vi "Current Loop 9505 (RT).vi"() -> ()   [LabVIEW 2012]
uses:
  <vilib>/LabVIEW Targets/FPGA/cRIO/cRIO-9505/controls.llb/_nicrio_cRIO-9505_DriveStatus.ctl
  <vilib>/addons/control/pid/pid.llb/PID (DBL).vi
  <vilib>/FPGAPlugInAG/cRIO-9074/niLvFpga_Open_cRIO-9074.vi
  <vilib>/Utility/error.llb/Error Cluster From Error Code.vi
  <vilib>/rvi/errors/niLvFpgaAdjustHostInterfaceError.vi
  <vilib>/FPGAPlugInAG/cRIO-9074/niLvFpga_Close_cRIO-9074.vi
  <vilib>/rvi/interface/nirviOpenFPGA/nirviOpenFPGA.xnode
  FPGA Bitfiles/DepthCtrlExperim_FPGATarget_CurrentLoop9505(_EF930710.lvbitx
  <vilib>/rvi/interface/nirviReadWriteControl/nirviReadWriteControl.xnode
  <vilib>/rvi/interface/nirviCloseFPGA/nirviCloseFPGA.xnode
  NiFpgaLv.dll
  <vilib>/addons/control/pid/NI_PID_pid.lvlib
panel:
  out "Time Response":cluster{"Actual Depth (m)":dbl, "setpoint":dbl}(graph)
  out "dt out (s)":dbl
  in  "Reinitialize? (F)":bool
  in  "output range":cluster{"output high":dbl, "output low":dbl}={"output high"=100.0, "output low"=-100.0}
  out "Ctrl Output":dbl
  in  "Sampling Time dt (s)":dbl
  in  "PID gains":T1={"proportional gain (Kc)"=1.0, "integral time (Ti, min)"=0.01, "derivative time (Td, min)"=0.0}
  in  "setpoint":dbl
  in  "Disable":bool
  in  "Disable":bool
  out "Loop Counter DEBUG":dbl
  out "Actual Depth DEBUG":dbl
  in  "Stop AutoTune":bool
  out "Actual Depth (m)":dbl(slide)
  in  "Switch To Autotune Output":bool
  in  "Enable":bool
  in  "Enable":bool
  out "Drive Status 2":T2
  out "Measured Current (Amps) 2":dbl
  in  "Current Loop Rate (usec) 2":u32=50
  in  "Drive Direction 2":enum16{"Clockwise", "Counterclockwise"}(ring)
  in  "Current Setpoint (Amps) 2":dbl(slide)
  in  "Current PI Gains 2":T3={"Proportional Gain"=20, "Integral Gain"=10, "Derivative Gain"=0}
  in  "Current Limit (Amps) 2":dbl=1.0
  in  "Current Limit (Amps)":dbl=1.0
  in  "Current PI Gains":T3={"Proportional Gain"=20, "Integral Gain"=10, "Derivative Gain"=0}
  in  "Current Setpoint (Amps)":dbl(slide)
  out "Measured Current (Amps)":dbl
  out "Drive Status":T2
  in  "Drive Direction":enum16{"Clockwise", "Counterclockwise"}(ring)
  in  "Current Loop Rate (usec)":u32=50
  in  "?":bool
  out "Raw Voltage":dbl(graph)
  out "error out 2":errorcluster
  in  "Wait ms":dbl
  in  "Density of Water":dbl
  in  "Atm Offset":dbl
  out "PSI":dbl(knob)
  out "PSI":dynamicdata(graph)
  out "Absolute Depth (m)":dbl(slide)
  in  "resource name":tag="RIO0::INSTR"
  out "error out":errorcluster
  in  "stop":bool
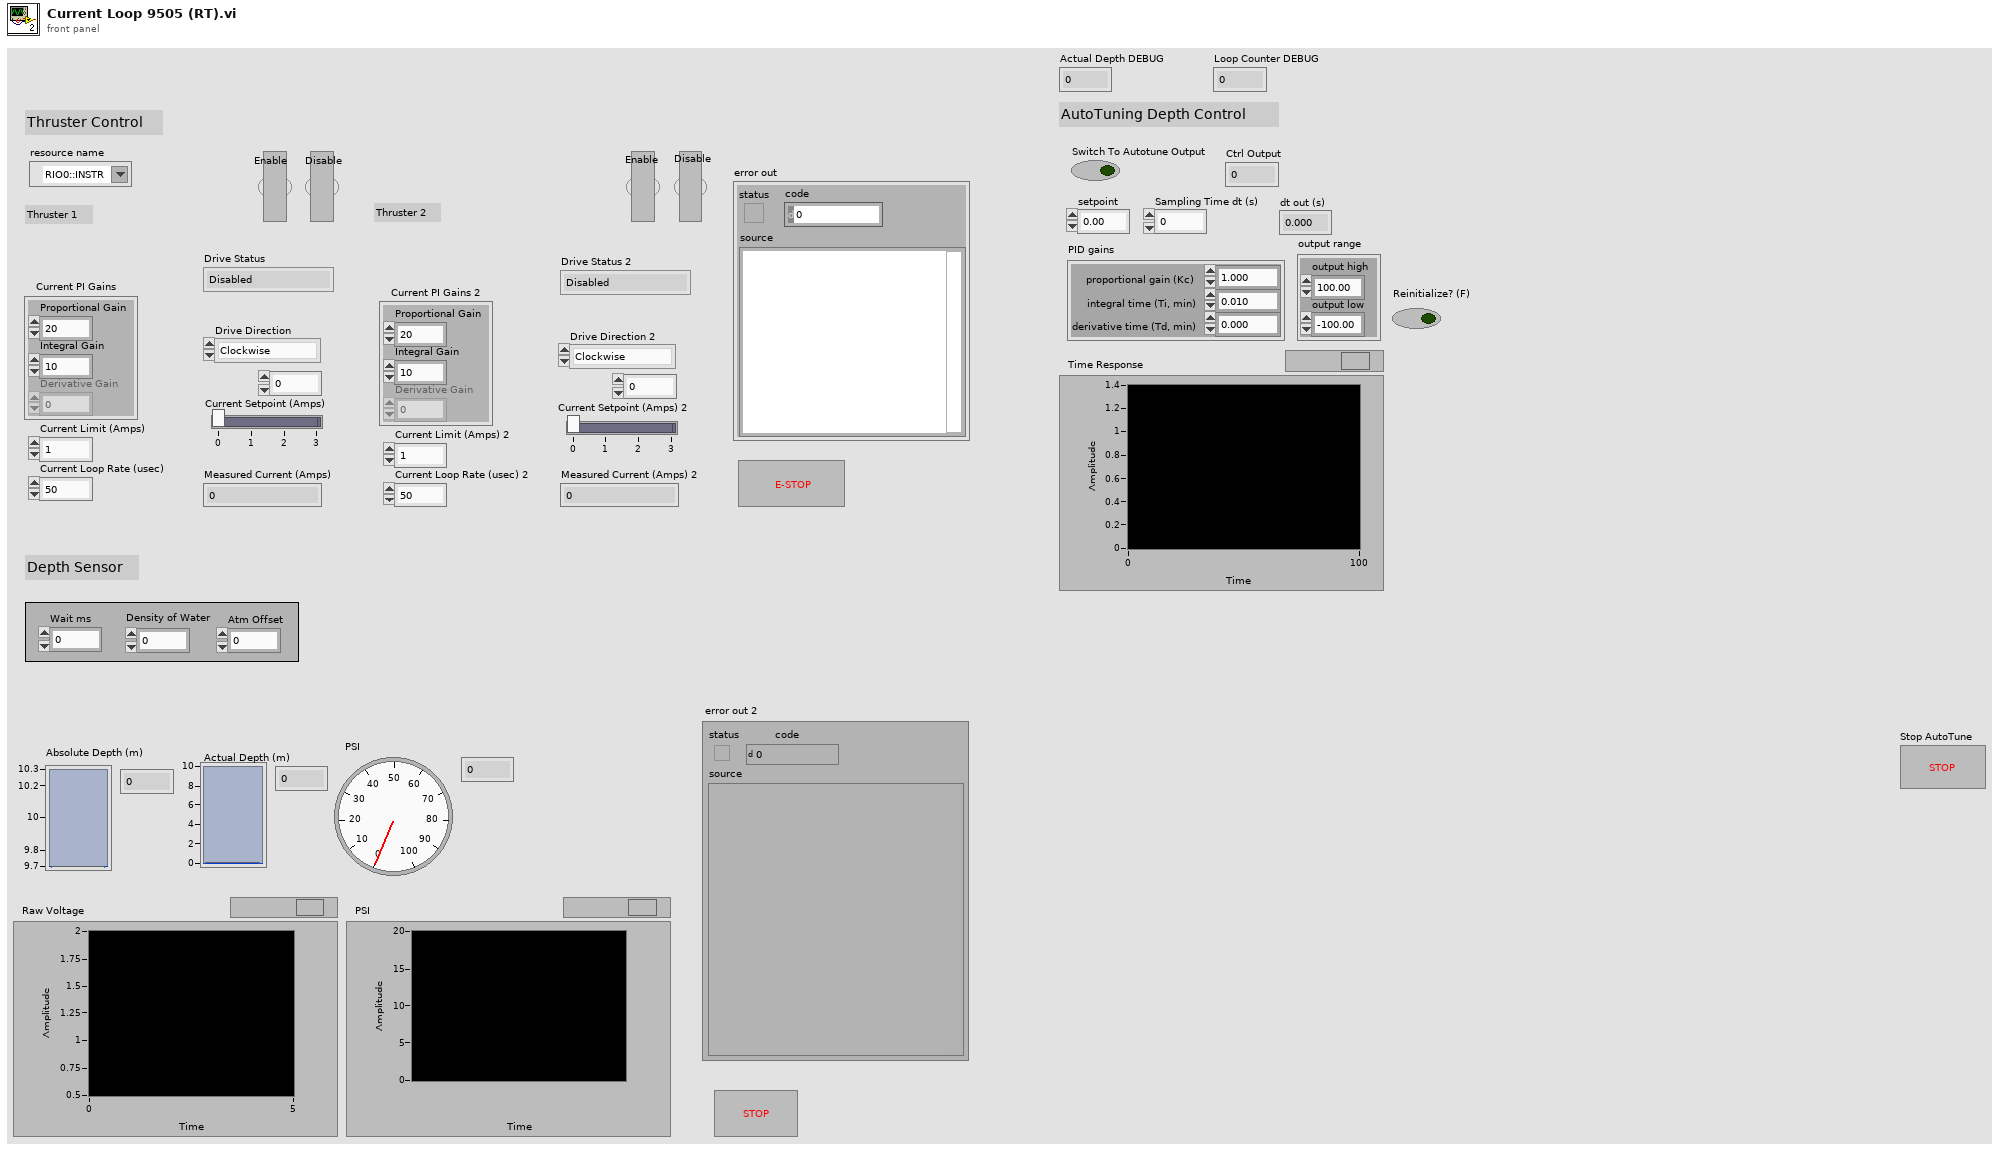
[diagram p1: front panel]
types:
  T1 = cluster{"proportional gain (Kc)":dbl, "integral time (Ti, min)":dbl, "derivative time (Td, min)":dbl}
  T2 = typedef "_nicrio_cRIO-9505_DriveStatus.ctl" = enum8{"Enabled", "Disabled", "Disabled by Drive Fault", "Disabled by Temp. Fault", "Disabled by E-Stop", "Unknown"}
  T3 = cluster{"Proportional Gain":i16, "Integral Gain":i16, "Derivative Gain":i16}
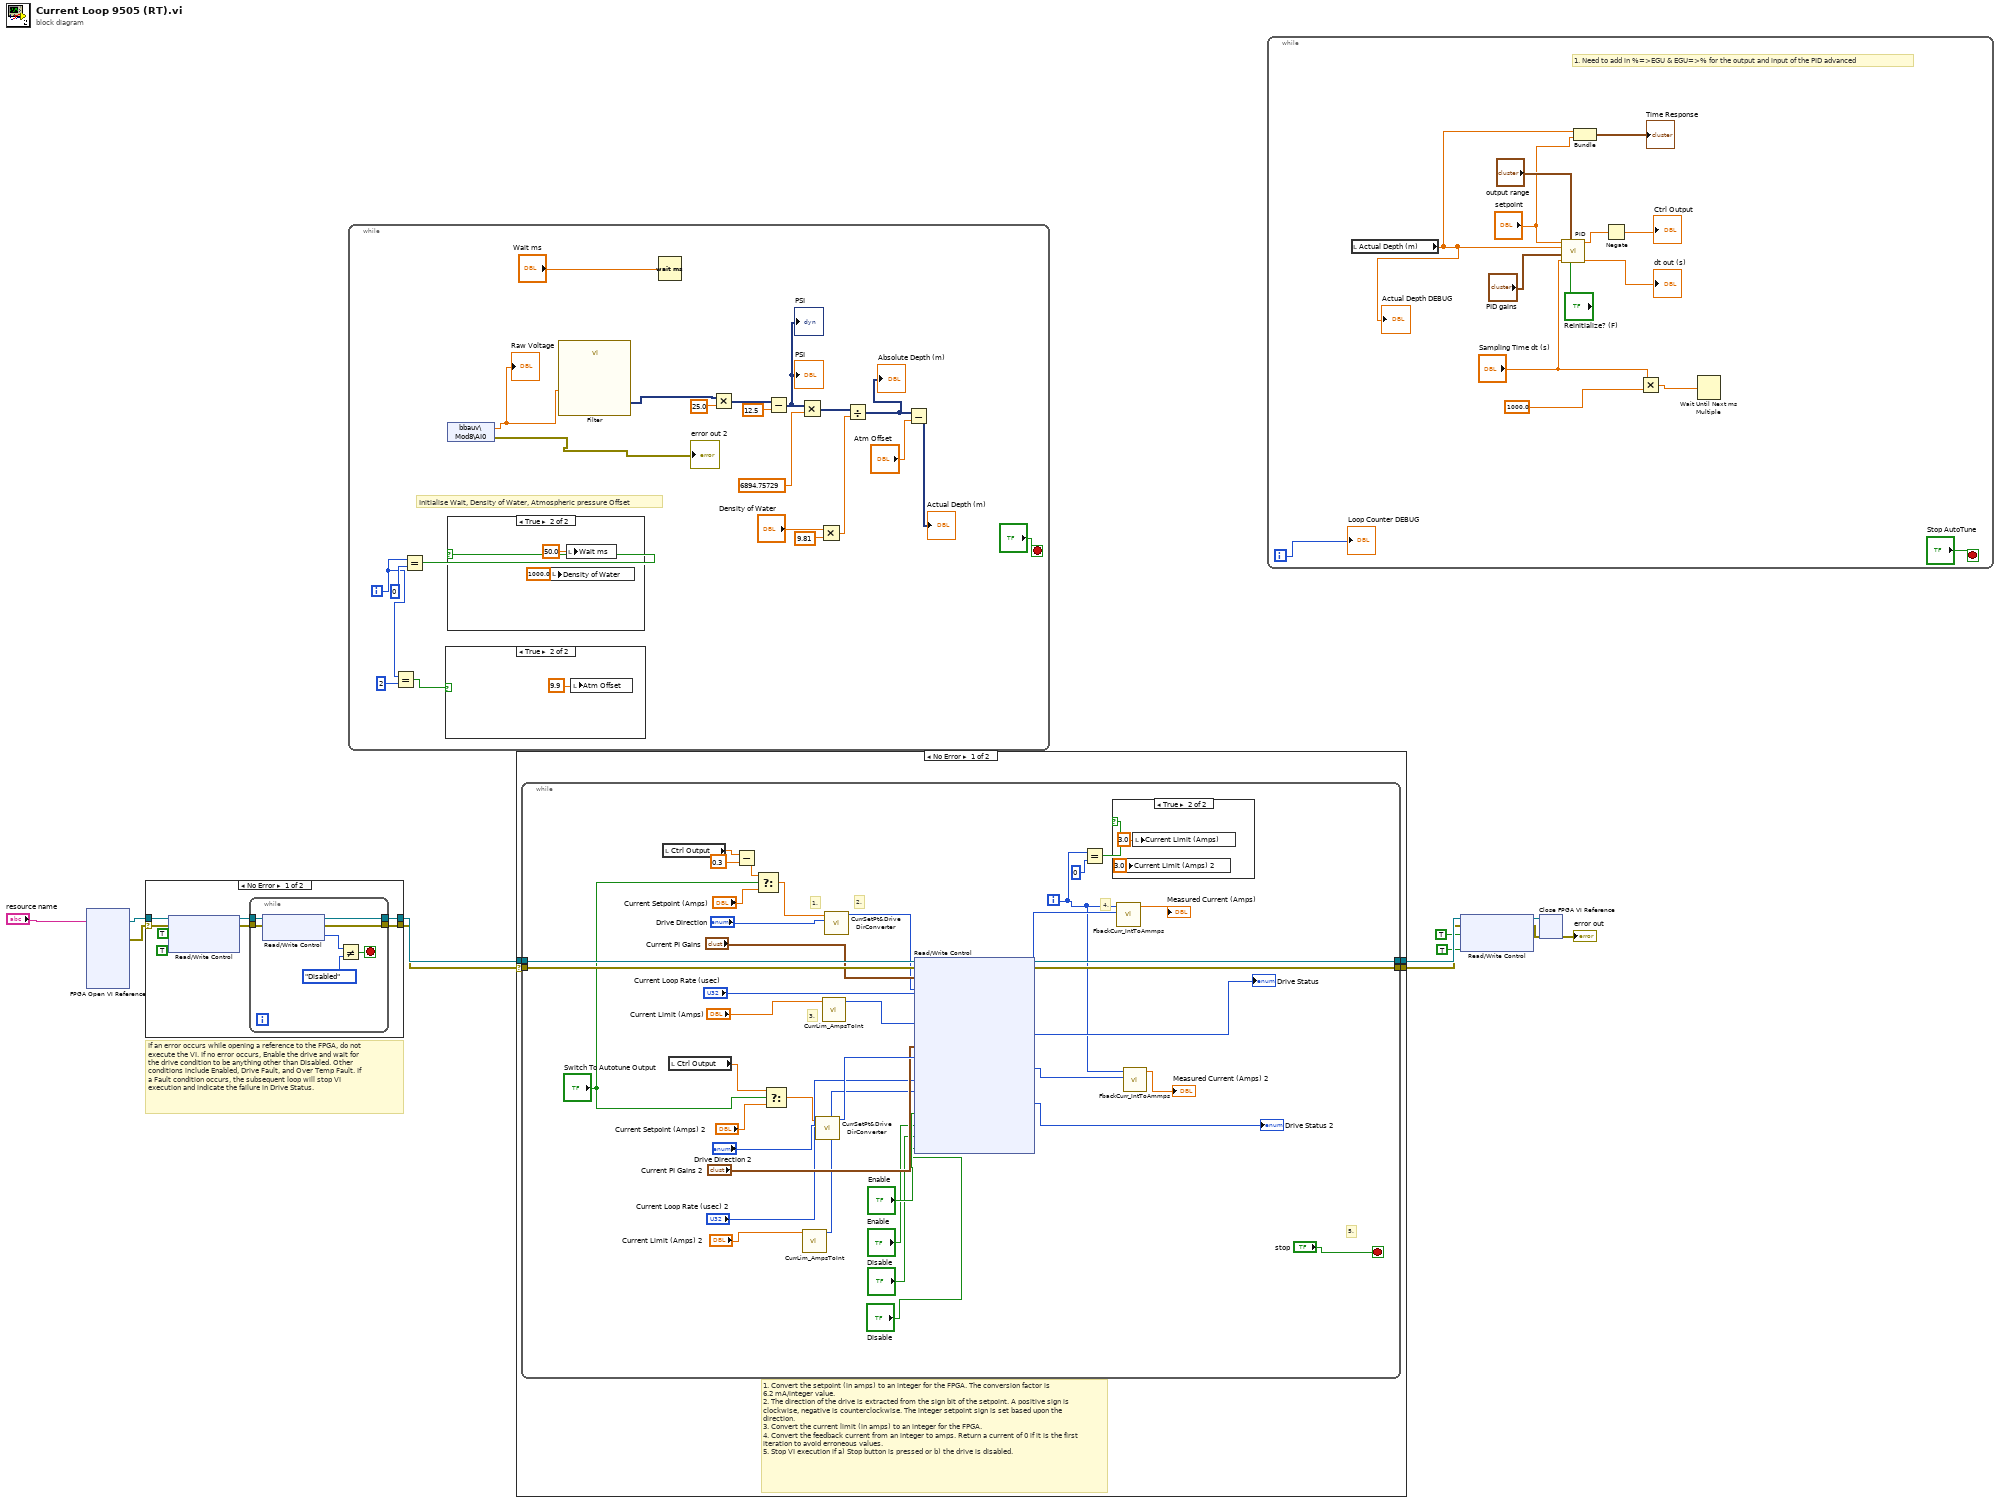
[diagram p0: block diagram]
diagram:
  # "If an error occurs while opening a reference to the FPGA, do not\nexecute the VI. If no error occurs, Enable the drive and wait for\nthe drive condition to be anything other than Disabled. Other\nconditions include Enabled, Drive Fault, and Over Temp Fault. If\na Fault condition occurs, the subsequent loop will stop VI\nexecution and indicate the failure in Drive Status."
  n1 = xnode "FPGA Open VI Reference"("resource name"="resource name") -> ("FPGA VI Reference Out"=w5:refnum<k20>, "error out"=w4:errorcluster)  [unwired: 1 in]
  n2 = case shown="No Error" w4 {
    selector: w4 -> [w15 w28]
    tunnel: w5 -> [w18 w29]
    tunnel: [w20 w29] -> w7
    tunnel: [w14 w28] -> w6
    frame No Error {
      n3 = xnode "Read/Write Control"("FPGA VI Reference In"=w18, "error in"=w15, "Enable Drive"=TRUE, "Enable Drive 2"=TRUE) -> ("FPGA VI Reference Out"=w17:refnum<k20>, "error out"=w16:errorcluster)
      n4 = while {
        tunnel: [w27] -> w20
        tunnel: w17 -> [w23]
        tunnel: w16 -> [w24]
        tunnel: [w21] -> w14
        stop <- w22 stop-if-true
        n5 = xnode "Read/Write Control"("FPGA VI Reference In"=w23, "error in"=w24) -> ("FPGA VI Reference Out"=w27:refnum<k20>, "error out"=w21:errorcluster, "Drive Status"=w26:T2)
        n6 = Not Equal?(x=w26, y=_nicrio_cRIO-9505_DriveStatus."Disabled") -> (x != y?=w22:bool)
      }
    }
    frame Error {
      # "Error occurred. Do not run."
    }
  }
  n7 = while {
    i -> [w36]
    stop <- "?" stop-if-true
    # "Initialise Wait, Density of Water, Atmospheric pressure Offset"
    n8 = Equal?(x=w36, y=2) -> (x = y?=w34:bool)
    n9 = Equal?(x=w36, y=0) -> (x = y?=w37:bool)
    n10 = case shown="True" w34 {
      frame False {
      }
      frame True {
        n11 = local write "Atm Offset"(9.9) -> ()
      }
    }
    n12 = shared-variable "bbauv\\Mod8\\AI0"() -> (w32:dbl, error out=→"error out 2":errorcluster)  [unwired: 1 in]
    "Raw Voltage" <- w32
    n13 = case shown="True" w37 {
      frame False {
      }
      frame True {
        n14 = local write "Density of Water"(1000.0) -> ()
        n15 = local write "Wait ms"(50.0) -> ()
      }
    }
    n16 = call "Filter"("Signal"=w32) -> ("Filtered Signal"=w33:dynamicdata)  [unwired: 9 in, 1 out]
    n17 = Wait (ms)(milliseconds to wait="Wait ms") -> ()  [unwired: 1 out]
    n18 = Multiply(x=w33, y=25.0) -> (x*y=w48:dynamicdata)
    n19 = Subtract(x=w48, y=12.5) -> (x-y=w41:dynamicdata)
    "PSI" <- w41
    "PSI" <- w41
    n20 = Multiply(x=w41, y=6894.75729) -> (x*y=w40:dynamicdata)
    n21 = Multiply(x="Density of Water", y=9.81) -> (x*y=w44:dbl)
    n22 = Divide(x=w40, y=w44) -> (x/y=w39:dynamicdata)
    "Absolute Depth (m)" <- w39
    n23 = Subtract(x=w39, y="Atm Offset") -> (x-y=→"Actual Depth (m)":dynamicdata)
  }
  n24 = case shown="No Error" w6 {
    selector: w6 -> [w55 w100]
    tunnel: [w58 w101] -> w12
    tunnel: [w57 w100] -> w11
    tunnel: w7 -> [w56 w101]
    frame No Error {
      # "1. Convert the setpoint (in amps) to an integer for the FPGA. The conversion factor is \n6.2 mA/integer value.\n2. The direction of the drive is extracted from the sign bit of the setpoint. A positive sign is clockwise, negative is counterclockwise. The integer setpoint sign is set based upon the direction.\n3. Convert the current limit (in amps) to an integer for the FPGA.\n4. Convert the feedback current from an integer to amps. Return a current of 0 if it is the first iteration to avoid erroneous values.\n5. Stop VI execution if a) Stop button is pressed or b) the drive is disabled."
      n25 = while {
        tunnel: w56 -> [w97]
        tunnel: [w95] -> w58
        tunnel: w55 -> [w96]
        tunnel: [w94] -> w57
        i -> [w64]
        stop <- "stop" stop-if-true
        # "2."
        # "1."
        # "5."
        # "4."
        # "3."
        n26 = local read "Ctrl Output"() -> (w61:dbl)
        n27 = local read "Ctrl Output"() -> (w69:dbl)
        n28 = Subtract(x=w61, y=0.3) -> (x-y=w59:dbl)
        n29 = Select(t=w59, s="Switch To Autotune Output", f="Current Setpoint (Amps)") -> (s? t:f=w70:dbl)
        n30 = Select(t=w69, s="Switch To Autotune Output", f="Current Setpoint (Amps) 2") -> (s? t:f=w73:dbl)
        n31 = call "CurrLim_AmpsToInt.vi"("Current Limit (Amps)"="Current Limit (Amps) 2") -> ("Numeric"=w75:i16)  [unwired: 10 in]
        n32 = call "CurrSetPt&DriveDirConverter.vi"("Drive Direction"="Drive Direction 2", "Current Setpoint (Amps)"=w73) -> ("Numeric"=w83:i16)  [unwired: 9 in]
        n33 = call "CurrLim_AmpsToInt.vi"("Current Limit (Amps)"="Current Limit (Amps)") -> ("Numeric"=w91:i16)  [unwired: 10 in]
        n34 = call "CurrSetPt&DriveDirConverter.vi"("Drive Direction"="Drive Direction", "Current Setpoint (Amps)"=w70) -> ("Numeric"=w89:i16)  [unwired: 9 in]
        n35 = xnode "Read/Write Control"("FPGA VI Reference In"=w97, "error in"=w96, "Current PI gains"="Current PI Gains", "Current Setpoint"=w89, "Current Loop Rate (usec)"="Current Loop Rate (usec)", "Current Limit"=w91, "Current PI gains 2"="Current PI Gains 2", "Current Setpoint 2"=w83, "Current Loop Rate (usec) 2"="Current Loop Rate (usec) 2", "Current Limit 2"=w75, "Enable Drive"="Enable", "Enable Drive 2"="Enable", "Disable Drive"="Disable", "Disable Drive 2"="Disable") -> ("FPGA VI Reference Out"=w95:refnum<k20>, "error out"=w94:errorcluster, "Current Feedback"=w86:i16, "Drive Status"=→"Drive Status":T2, "Current Feedback 2"=w77:i16, "Drive Status 2"=→"Drive Status 2":T2)
        n36 = Equal?(x=w64, y=0) -> (x = y?=w62:bool)
        n37 = case shown="True" w62 {
          frame False {
          }
          frame True {
            n38 = local write "Current Limit (Amps) 2"(3.0) -> ()
            n39 = local write "Current Limit (Amps)"(3.0) -> ()
          }
        }
        n40 = call "FbackCurr_IntToAmmps.vi"("Current Feedback"=w86, "Numeric"=w64) -> ("Measured Current (Amps)"=→"Measured Current (Amps)":dbl)  [unwired: 9 in]
        n41 = call "FbackCurr_IntToAmmps.vi"("Current Feedback"=w77, "Numeric"=w64) -> ("Measured Current (Amps)"=→"Measured Current (Amps) 2":dbl)  [unwired: 9 in]
      }
    }
    frame Error {
      # "Error occurred. Do not run."
    }
  }
  n42 = while {
    i -> [w114]
    stop <- "Stop AutoTune" stop-if-true
    # "1. Need to add in %=>EGU & EGU=>% for the output and input of the PID advanced"
    n43 = local read "Actual Depth (m)"() -> (w103:dbl)
    "Actual Depth DEBUG" <- w103
    n44 = call-poly <vilib>:"PID.vi"("reinitialize? (F)"="Reinitialize? (F)", "output range"="output range", "dt (s)"="Sampling Time dt (s)", "PID gains"="PID gains", "process variable"=w103, "setpoint"="setpoint") -> ("dt out (s)"=→"dt out (s)":dbl, "output"=w105:dbl)  [unwired: 4 in]
    n45 = Bundle("Actual Depth (m)"=w103, "setpoint"="setpoint") -> (→"Time Response":cluster{"Actual Depth (m)":dbl, "setpoint":dbl})  [unwired: 1 in]
    n46 = Negate(x=w105) -> (-x=→"Ctrl Output":dbl)
    n47 = Multiply(x="Sampling Time dt (s)", y=1000.0) -> (x*y=w112:dbl)
    n48 = Wait Until Next ms Multiple(millisecond multiple=w112) -> ()  [unwired: 1 out]
    "Loop Counter DEBUG" <- w114
  }
  n49 = xnode "Read/Write Control"("FPGA VI Reference In"=w12, "error in"=w11, "Disable Drive"=TRUE, "Disable Drive 2"=TRUE) -> ("FPGA VI Reference Out"=w9:refnum<k20>, "error out"=w8:errorcluster)
  n50 = xnode "Close FPGA VI Reference"("FPGA VI Reference In"=w9, "error in"=w8) -> ("error out"=→"error out":errorcluster)
